vi "build wave.vi"() -> (2 "数组":waveform(dbl)[](array[waveform]))   [LabVIEW 2009]
uses:
  <vilib>/measure/NI_MABase.lvlib
panel:
  in  "fs":i32=1000
  in  "reads":i32=1000
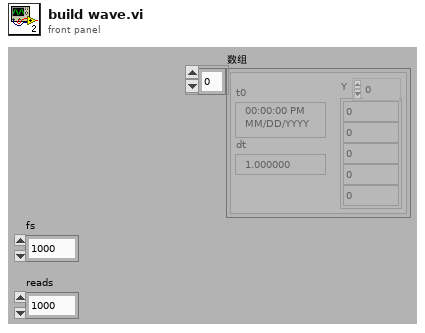
[diagram p1: front panel]
types:
  T1 = enum16{"Sine Wave", "Triangle Wave", "Square Wave", "Sawtooth Wave"}
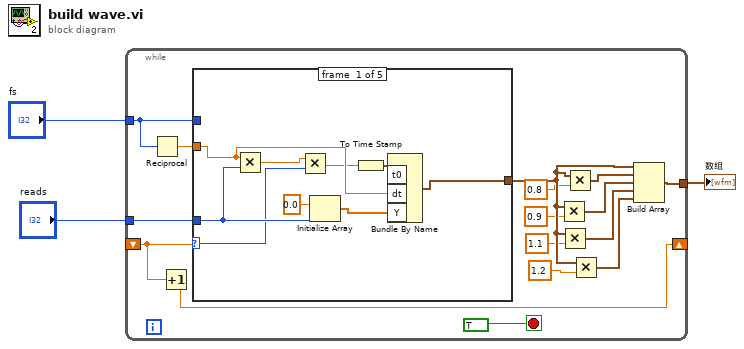
[diagram p0: block diagram]
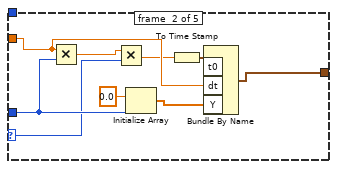
[diagram p2: hidden frame]
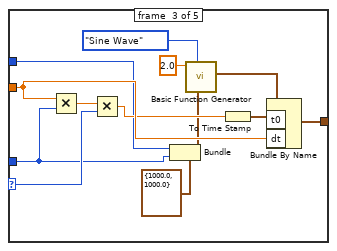
[diagram p3: hidden frame]
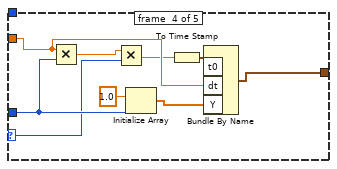
[diagram p4: hidden frame]
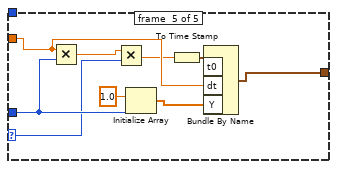
[diagram p5: hidden frame]
diagram:
  n1 = while {
    tunnel: "reads" -> [w18]
    tunnel: [w8] -> w2
    tunnel: "fs" -> [w6]
    shift-right: [w5] -> _
    shift-left: _ -> [w4]
    stop <- TRUE stop-if-true
    n2 = Reciprocal(x=w6) -> (1/x=w7:dbl)
    n3 = Increment(x=w4) -> (x+1=w5:dbl)
    n4 = case shown="2" w4 {
      selector: w4 -> [w23 w32 w49 w54 w63]
      tunnel: w18 -> [w25 w34 w39 w56 w65]
      tunnel: [w26 w35 w45 w57 w66] -> w13
      tunnel: w7 -> [w22 w31 w48 w53 w62]
      tunnel: w6 -> [_ _ w40 _ _]
      frame #0 {
        n5 = Multiply(x=w22, y=w25) -> (x*y=w24:dbl)
        n6 = Multiply(x=w24, y=w23) -> (x*y=w21:dbl)
        n7 = Initialize Array(0.0 ("元素"), w25) -> (w27:dbl[])
        n8 = To Time Stamp(1:w21) -> (0:w20:timestamp)
        n9 = Bundle By Name("t0"=w20, "dt"=w22, "Y"=w27) -> (w26:waveform(dbl))  [unwired: 1 out]
      }
      frame #1 {
        n10 = Multiply(x=w31, y=w34) -> (x*y=w33:dbl)
        n11 = Multiply(x=w33, y=w32) -> (x*y=w30:dbl)
        n12 = Initialize Array(0.0 ("元素"), w34) -> (w36:dbl[])
        n13 = To Time Stamp(1:w30) -> (0:w29:timestamp)
        n14 = Bundle By Name("t0"=w29, "dt"=w31, "Y"=w36) -> (w35:waveform(dbl))  [unwired: 1 out]
      }
      frame #2 {
        n15 = Multiply(x=w48, y=w39) -> (x*y=w50:dbl)
        n16 = Multiply(x=w50, y=w49) -> (x*y=w47:dbl)
        n17 = Bundle(cluster=cluster{"Fs":dbl, "#s":dbl} {"Fs"=1000.0, "#s"=1000.0} ("sampling info"), "Fs"=w40, "#s"=w39) -> (w41:cluster{"Fs":dbl, "#s":dbl})
        n18 = call <vilib>:"Basic Function Generator.vi"("sampling info"=w41, "signal type"=T1."Sine Wave", "frequency"=2.0) -> ("signal out"=w44:waveform(dbl))  [unwired: 6 in, 2 out]
        n19 = To Time Stamp(1:w47) -> (0:w46:timestamp)
        n20 = Bundle By Name(cluster=w44, "t0"=w46, "dt"=w48) -> (w45:waveform(dbl))
      }
      frame #3 {
        n21 = Multiply(x=w53, y=w56) -> (x*y=w55:dbl)
        n22 = Multiply(x=w55, y=w54) -> (x*y=w52:dbl)
        n23 = Initialize Array(1.0 ("元素"), w56) -> (w58:dbl[])
        n24 = To Time Stamp(1:w52) -> (0:w51:timestamp)
        n25 = Bundle By Name("t0"=w51, "dt"=w53, "Y"=w58) -> (w57:waveform(dbl))  [unwired: 1 out]
      }
      frame #4 {
        n26 = Multiply(x=w62, y=w65) -> (x*y=w64:dbl)
        n27 = Multiply(x=w64, y=w63) -> (x*y=w61:dbl)
        n28 = Initialize Array(1.0 ("元素"), w65) -> (w67:dbl[])
        n29 = To Time Stamp(1:w61) -> (0:w60:timestamp)
        n30 = Bundle By Name("t0"=w60, "dt"=w62, "Y"=w67) -> (w66:waveform(dbl))  [unwired: 1 out]
      }
    }
    n31 = Multiply(x=w13, y=0.9) -> (x*y=w16:waveform(dbl))
    n32 = Multiply(x=w13, y=1.1) -> (x*y=w15:waveform(dbl))
    n33 = Multiply(x=w13, y=0.8) -> (x*y=w17:waveform(dbl))
    n34 = Multiply(x=w13, y=1.2) -> (x*y=w14:waveform(dbl))
    n35 = Build Array(w13, w17, w16, w15, w14) -> (w8:waveform(dbl)[])
  }
  "数组" <- w2
